vi "FUG_PowerSupply.ProcCases.vi"(0 "i ref in":refnum<vi>, 1 "selector":string, 2 "Data":T1, 3 "call cluster":T2={"Object"="", "Selector"="", "CallType"=enum."synchronous", "Async Object"="", "Async Selector"="", "Data Descriptor"="", "Data"=[], "Error #"=0, "Expire"=0}, 5 "error in (no error)":errorcluster) -> (14 "i ref out":refnum<vi>, 17 "answer cluster":T2={"Object"="", "Selector"="", "CallType"=enum."synchronous", "Async Object"="", "Async Selector"="", "Data Descriptor"="", "Data"=[], "Error #"=0, "Expire"=0}, 19 "error out":errorcluster)   [LabVIEW 2014, in "FUG_PowerSupply.lvlib"]
doc: "This method is called by a process from within the default case in the event loop. The methods of a class that are linked to events will be called from THIS method. Add your code here."
uses:
  FUG_PowerSupply.lvlib
  CS_Core/CSSystem/CoreDefs/CoreDefs.call_type.ctl
  CS_Core/BaseProcess/BaseProcess.descriptor string definition.ctl
  CS_Core/CSSystem/CoreDefs/CoreDefs.rawDataType.ctl
  CS_Core/CSSystem/CoreLib/CoreLib.byte array 2 short.vi
  CS_Core/CSSystem/CoreLib/CoreLib.byte array 2 int.vi
  CS_Core/CSSystem/CoreLib/CoreLib.string 2 byte array.vi
  CS_Core/CSSystem/CoreLib/CoreLib.byte array 2 double.vi
  CS_Core/CSSystem/CoreLib/CoreLib.lvlib
  CS_Core/BaseProcess/BaseProcess.lvlib
  CS_Core/CAEObj/CAEObj.lvlib
  CS_Core/CSApplicationBaseClasses/PSChannelBase/PSChannelBase.lvlib
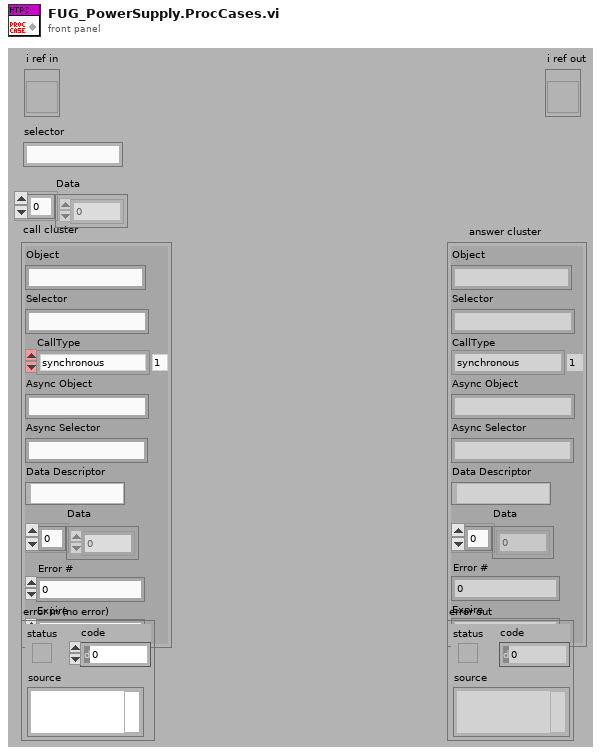
[diagram p1: front panel]
types:
  T1 = typedef "CoreDefs.rawDataType.ctl" = i8[]
  T2 = typedef "CoreDefs.call_type.ctl" = cluster{"Object":string, "Selector":string, "CallType":enum16{"simple", "synchronous", "asynchronous"}, "Async Object":string, "Async Selector":string, "Data Descriptor":T3, "Data":T1, "Error #":i32, "Expire":u32}
  T3 = typedef "BaseProcess.lvlib/BaseProcess.descriptor string definition.ctl" = string
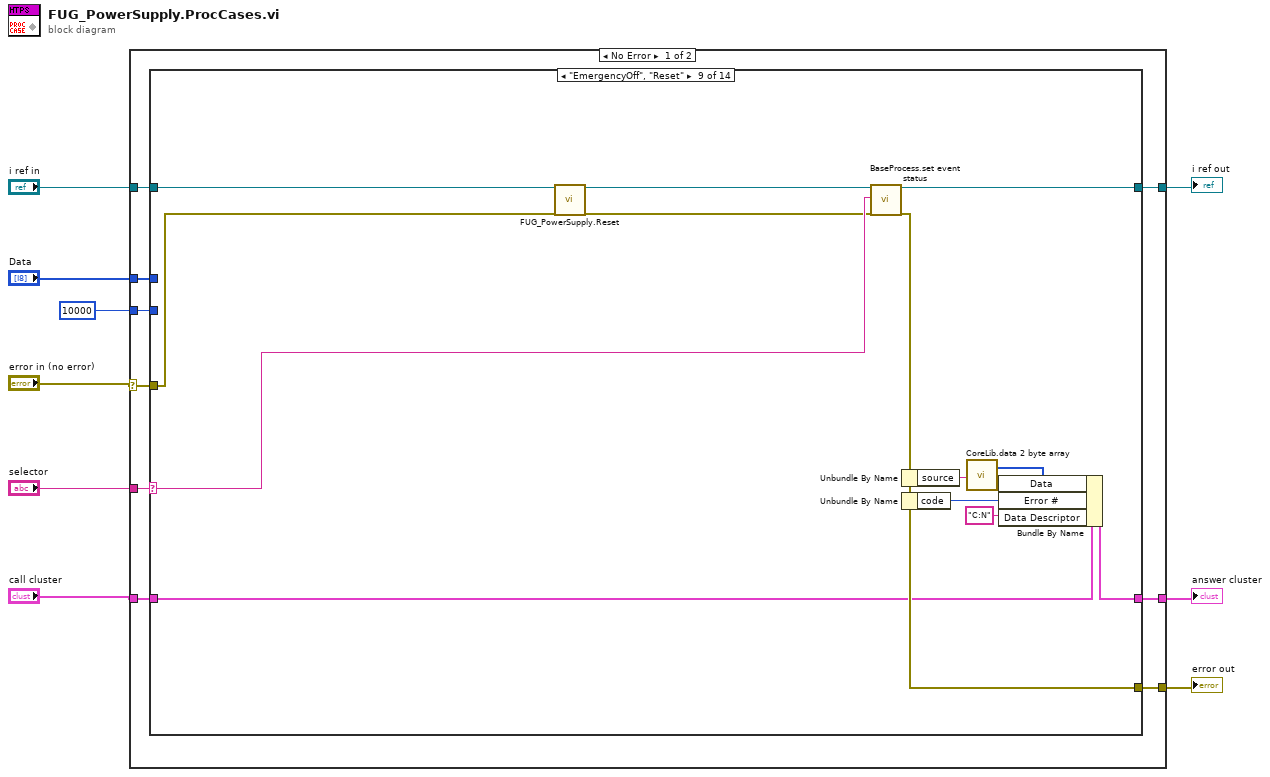
[diagram p0: block diagram]
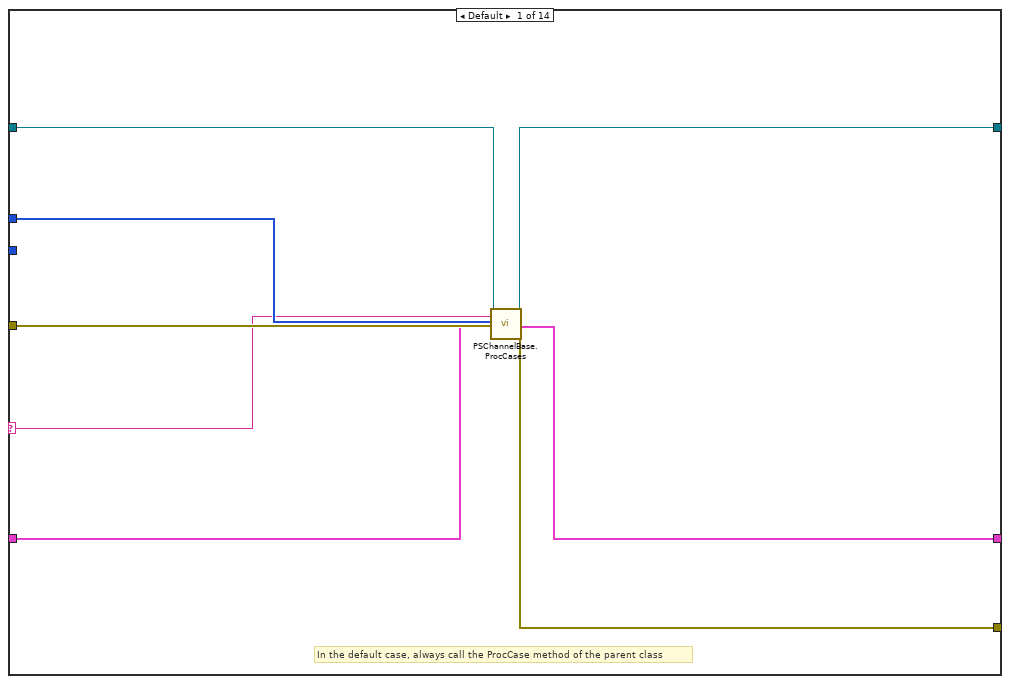
[diagram p2: hidden frame]
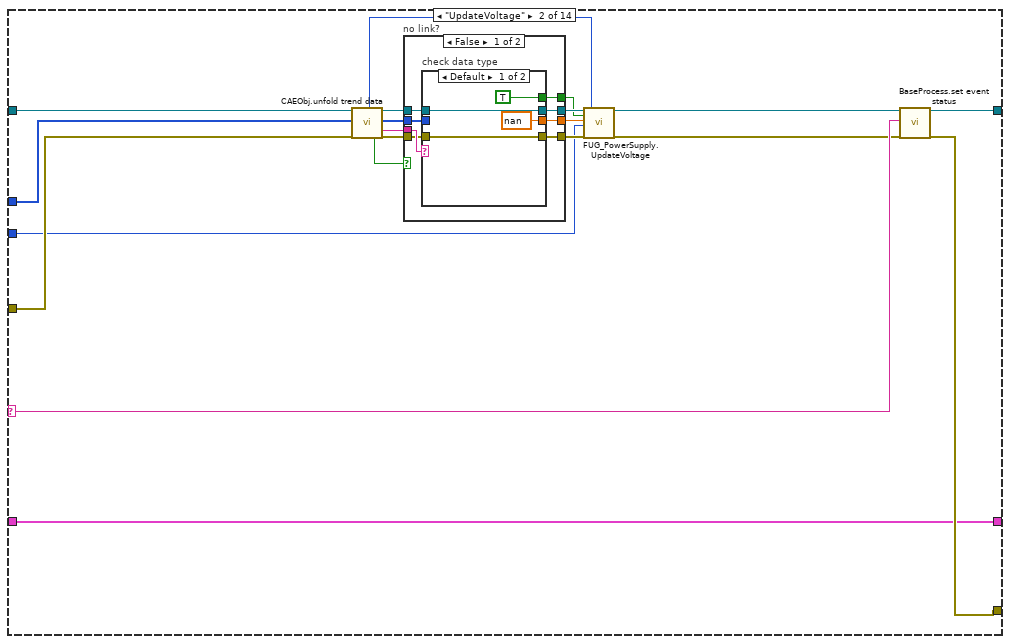
[diagram p3: hidden frame]
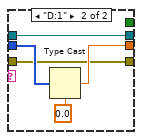
[diagram p4: hidden frame]
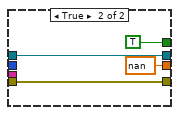
[diagram p5: hidden frame]
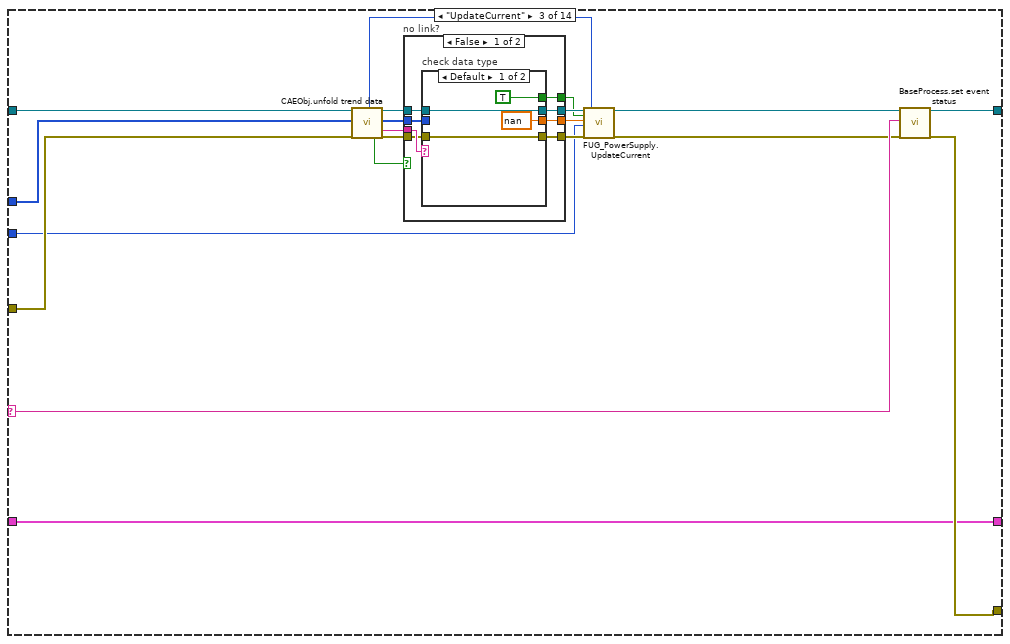
[diagram p6: hidden frame]
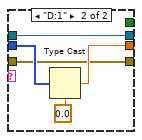
[diagram p7: hidden frame]
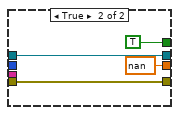
[diagram p8: hidden frame]
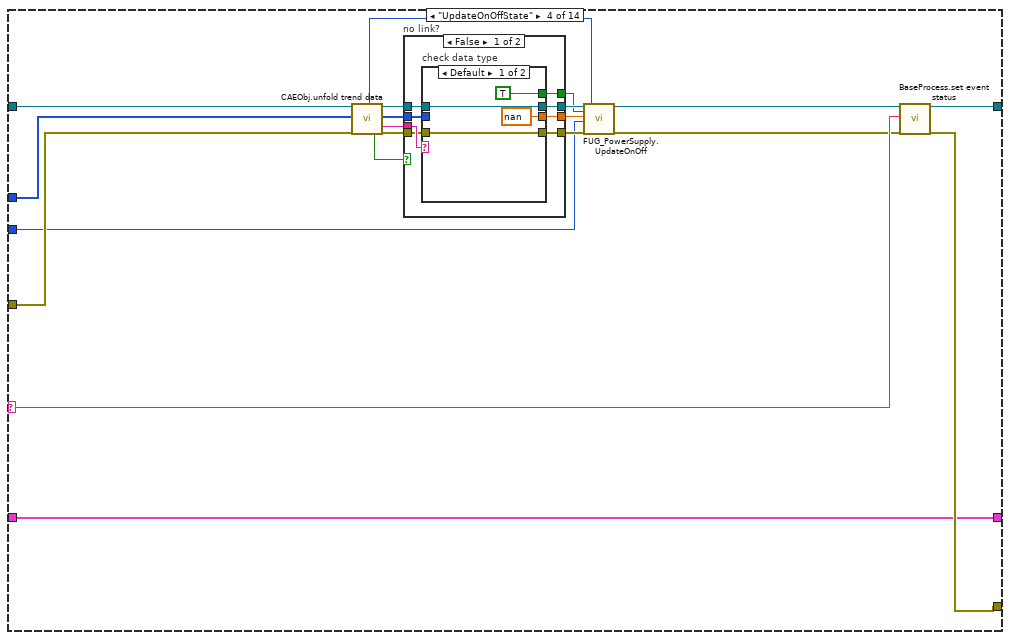
[diagram p9: hidden frame]
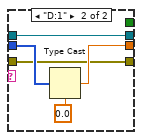
[diagram p10: hidden frame]
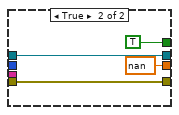
[diagram p11: hidden frame]
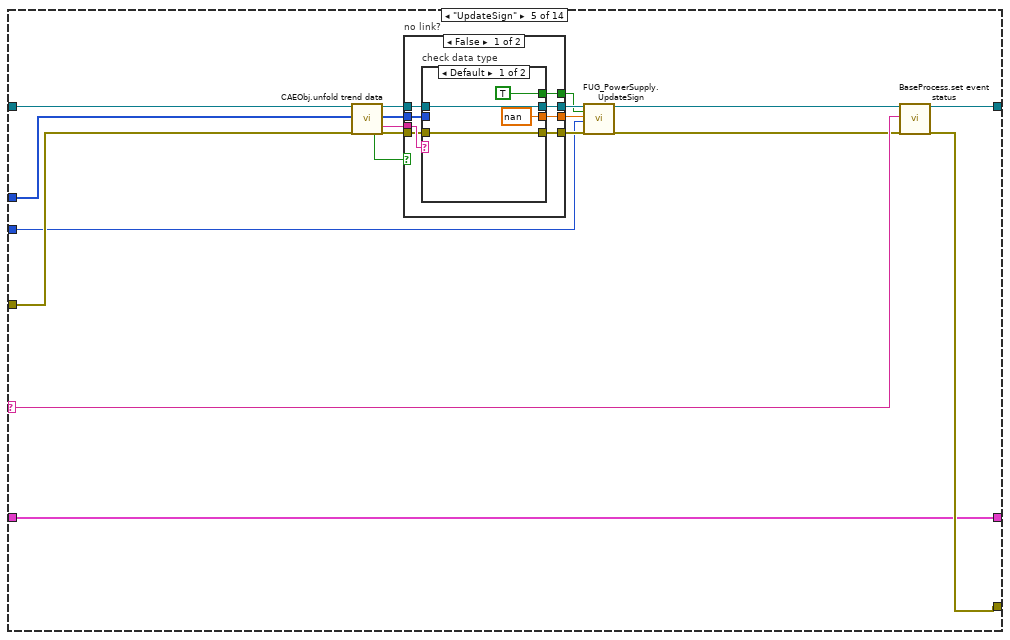
[diagram p12: hidden frame]
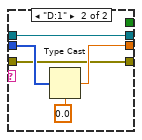
[diagram p13: hidden frame]
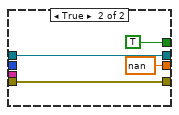
[diagram p14: hidden frame]
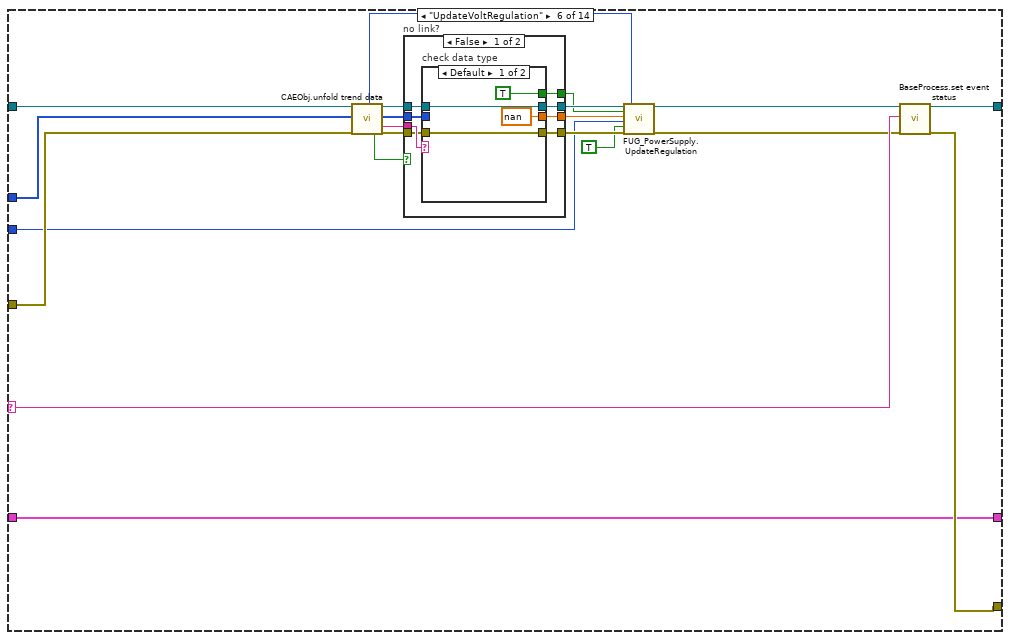
[diagram p15: hidden frame]
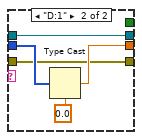
[diagram p16: hidden frame]
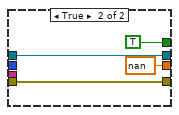
[diagram p17: hidden frame]
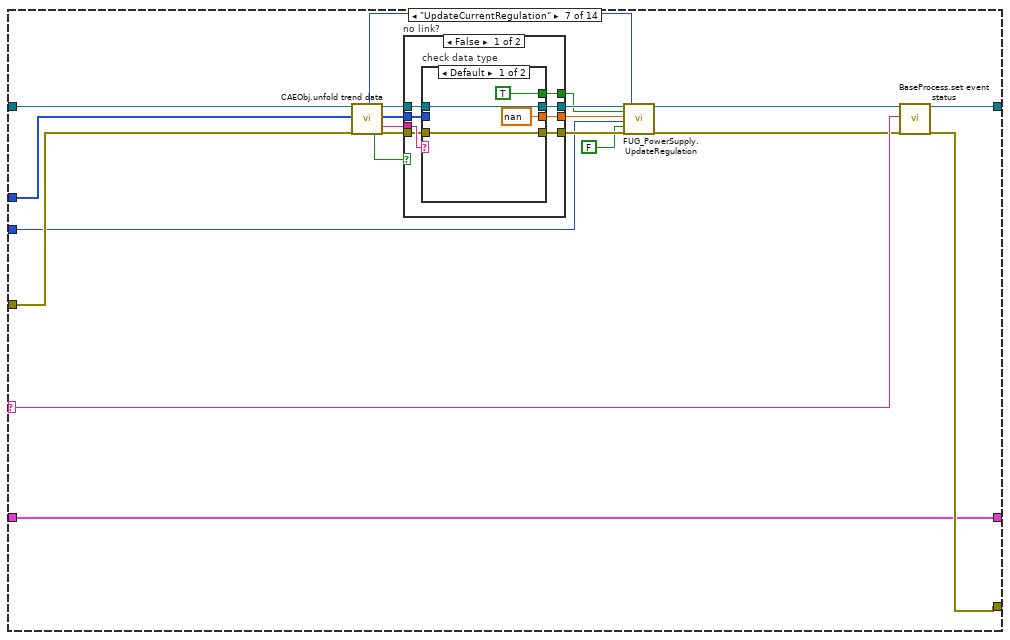
[diagram p18: hidden frame]
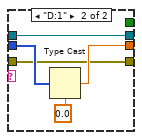
[diagram p19: hidden frame]
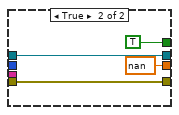
[diagram p20: hidden frame]
diagram:
  n1 = case shown="No Error" "error in (no error)" {
    selector: "error in (no error)" -> [w11 w453]
    tunnel: "selector" -> [w18 _]
    tunnel: [w17 w454] -> w3
    tunnel: "Data" -> [w16 _]
    tunnel: "call cluster" -> [w15 w454]
    tunnel: "i ref in" -> [w14 w455]
    tunnel: [w13 w455] -> w4
    tunnel: [w12 w453] -> w2
    tunnel: 10000 ("ms timeout (100)") -> [w10 _]
    frame No Error {
      n2 = case shown="\"EmergencyOff\", \"Reset\"" w18 {
        selector: w18 -> [w20 w40 w81 w122 w162 w204 w246 w285 w310 w328 w356 w386 w409 w435]
        tunnel: w16 -> [w21 w41 w82 w123 w163 w205 w247 _ _ _ _ _ _ _]
        tunnel: w14 -> [w19 w43 w84 w125 w165 w207 w249 w289 w312 w332 w360 w390 w411 w437]
        tunnel: [w26 w45 w86 w127 w167 w209 w251 w290 w313 w333 w361 w391 w414 w440] -> w13
        tunnel: w15 -> [w22 w44 w85 w126 w166 w208 w250 w277 w302 w321 w346 w377 w406 w433]
        tunnel: [w23 w44 w85 w126 w166 w208 w250 w280 w304 w323 w351 w381 w406 w433] -> w17
        tunnel: w11 -> [w25 w42 w83 w124 w164 w206 w248 w274 w301 w318 w345 w376 w403 w430]
        tunnel: [w24 w46 w87 w128 w168 w210 w252 w279 w303 w322 w350 w380 w413 w439] -> w12
        tunnel: w10 -> [_ w27 w68 w109 w150 w192 w234 _ _ _ _ _ _ _]
        frame Default {
          # "In the default case, always call the ProcCase method of the parent class"
          n3 = call "PSChannelBase.ProcCases.vi"("i ref in"=w19, "selector"=w20, "Data"=w21, "call cluster"=w22, "error in (no error)"=w25) -> ("i ref out"=w26:refnum<vi>, "answer cluster"=w23:T2, "error out"=w24:errorcluster)  [unwired: 12 in]
        }
        frame "UpdateVoltage" {
          n4 = call "CAEObj.unfold trend data.vi"("i ref in"=w43, "raw trend data"=w41, "error in (no error)"=w42) -> ("quality"=w28:i32, "no link"=w35:bool, "i ref out"=w39:refnum<vi>, "data"=w37:i8[], "typeDescriptor"=w36:string, "error out"=w38:errorcluster)  [unwired: 8 in, 3 out]
          n5 = case "no link?" shown="False" w35 {
            tunnel: [w54 w66] -> w34
            tunnel: [w53 w65] -> w33
            tunnel: w37 -> [w52 _]
            tunnel: w39 -> [w51 w66]
            tunnel: w36 -> [w50 _]
            tunnel: w38 -> [w49 w65]
            tunnel: [w48 TRUE ("badValue")] -> w30
            tunnel: [w47 nan] -> w29
            frame False {
              n6 = case "check data type" shown="Default" w50 {
                tunnel: [w56 w59] -> w54
                tunnel: [w57 w60] -> w53
                tunnel: w52 -> [_ w63]
                tunnel: w51 -> [w56 w59]
                tunnel: w49 -> [w57 w60]
                tunnel: [TRUE ("badValue") _] -> w48
                tunnel: [nan w61] -> w47
                frame Default {
                }
                frame "D:1" {
                  n7 = Type Cast(type=0.0, x=w63) -> (*(type *) &x=w61:dbl)
                }
              }
            }
            frame True {
            }
          }
          n8 = call "FUG_PowerSupply.UpdateVoltage.vi"("i ref in"=w34, "badValue"=w30, "moduleValue"=w29, "ms timeout (10000)"=w27, "error in (no error)"=w33, "voltageQuality"=w28) -> ("i ref out"=w32:refnum<vi>, "error out"=w31:errorcluster)  [unwired: 11 in, 1 out]
          n9 = call "BaseProcess.set event status.vi"("i ref in"=w32, "EventStatus"=w40, "error in (no error)"=w31) -> ("i ref out"=w45:refnum<vi>, "error out"=w46:errorcluster)  [unwired: 14 in, 1 out]
        }
        frame "UpdateCurrent" {
          n10 = call "CAEObj.unfold trend data.vi"("i ref in"=w84, "raw trend data"=w82, "error in (no error)"=w83) -> ("quality"=w69:i32, "no link"=w76:bool, "i ref out"=w80:refnum<vi>, "data"=w78:i8[], "typeDescriptor"=w77:string, "error out"=w79:errorcluster)  [unwired: 8 in, 3 out]
          n11 = case "no link?" shown="False" w76 {
            tunnel: [w95 w107] -> w75
            tunnel: [w94 w106] -> w74
            tunnel: w78 -> [w93 _]
            tunnel: w80 -> [w92 w107]
            tunnel: w77 -> [w91 _]
            tunnel: w79 -> [w90 w106]
            tunnel: [w89 TRUE ("badValue")] -> w71
            tunnel: [w88 nan] -> w70
            frame False {
              n12 = case "check data type" shown="Default" w91 {
                tunnel: [w97 w100] -> w95
                tunnel: [w98 w101] -> w94
                tunnel: w93 -> [_ w104]
                tunnel: w92 -> [w97 w100]
                tunnel: w90 -> [w98 w101]
                tunnel: [TRUE ("badValue") _] -> w89
                tunnel: [nan w102] -> w88
                frame Default {
                }
                frame "D:1" {
                  n13 = Type Cast(type=0.0, x=w104) -> (*(type *) &x=w102:dbl)
                }
              }
            }
            frame True {
            }
          }
          n14 = call "FUG_PowerSupply.UpdateCurrent.vi"("i ref in"=w75, "badValue"=w71, "moduleValue"=w70, "ms timeout (10000)"=w68, "error in (no error)"=w74, "quality"=w69) -> ("i ref out"=w73:refnum<vi>, "error out"=w72:errorcluster)  [unwired: 11 in, 1 out]
          n15 = call "BaseProcess.set event status.vi"("i ref in"=w73, "EventStatus"=w81, "error in (no error)"=w72) -> ("i ref out"=w86:refnum<vi>, "error out"=w87:errorcluster)  [unwired: 14 in, 1 out]
        }
        frame "UpdateOnOffState" {
          n16 = call "CAEObj.unfold trend data.vi"("i ref in"=w125, "raw trend data"=w123, "error in (no error)"=w124) -> ("quality"=w110:i32, "no link"=w117:bool, "i ref out"=w121:refnum<vi>, "data"=w119:i8[], "typeDescriptor"=w118:string, "error out"=w120:errorcluster)  [unwired: 8 in, 3 out]
          n17 = case "no link?" shown="False" w117 {
            tunnel: [w136 w148] -> w116
            tunnel: [w135 w147] -> w115
            tunnel: w119 -> [w134 _]
            tunnel: w121 -> [w133 w148]
            tunnel: w118 -> [w132 _]
            tunnel: w120 -> [w131 w147]
            tunnel: [w130 TRUE ("badValue")] -> w112
            tunnel: [w129 nan] -> w111
            frame False {
              n18 = case "check data type" shown="Default" w132 {
                tunnel: [w138 w141] -> w136
                tunnel: [w139 w142] -> w135
                tunnel: w134 -> [_ w145]
                tunnel: w133 -> [w138 w141]
                tunnel: w131 -> [w139 w142]
                tunnel: [TRUE ("badValue") _] -> w130
                tunnel: [nan w143] -> w129
                frame Default {
                }
                frame "D:1" {
                  n19 = Type Cast(type=0.0, x=w145) -> (*(type *) &x=w143:dbl)
                }
              }
            }
            frame True {
            }
          }
          n20 = call "FUG_PowerSupply.UpdateOnOff.vi"("i ref in"=w116, "badValue"=w112, "moduleValue"=w111, "ms timeout (10000)"=w109, "error in (no error)"=w115, "onOffQuality"=w110) -> ("i ref out"=w114:refnum<vi>, "error out"=w113:errorcluster)  [unwired: 11 in, 1 out]
          n21 = call "BaseProcess.set event status.vi"("i ref in"=w114, "EventStatus"=w122, "error in (no error)"=w113) -> ("i ref out"=w127:refnum<vi>, "error out"=w128:errorcluster)  [unwired: 14 in, 1 out]
        }
        frame "UpdateSign" {
          n22 = call "CAEObj.unfold trend data.vi"("i ref in"=w165, "raw trend data"=w163, "error in (no error)"=w164) -> ("no link"=w157:bool, "i ref out"=w161:refnum<vi>, "data"=w159:i8[], "typeDescriptor"=w158:string, "error out"=w160:errorcluster)  [unwired: 8 in, 4 out]
          n23 = case "no link?" shown="False" w157 {
            tunnel: [w176 w188] -> w156
            tunnel: [w175 w187] -> w155
            tunnel: w159 -> [w174 _]
            tunnel: w161 -> [w173 w188]
            tunnel: w158 -> [w172 _]
            tunnel: w160 -> [w171 w187]
            tunnel: [w170 TRUE ("badValue")] -> w152
            tunnel: [w169 nan] -> w151
            frame False {
              n24 = case "check data type" shown="Default" w172 {
                tunnel: [w178 w181] -> w176
                tunnel: [w179 w182] -> w175
                tunnel: w174 -> [_ w185]
                tunnel: w173 -> [w178 w181]
                tunnel: w171 -> [w179 w182]
                tunnel: [TRUE ("badValue") _] -> w170
                tunnel: [nan w183] -> w169
                frame Default {
                }
                frame "D:1" {
                  n25 = Type Cast(type=0.0, x=w185) -> (*(type *) &x=w183:dbl)
                }
              }
            }
            frame True {
            }
          }
          n26 = call "FUG_PowerSupply.UpdateSign.vi"("i ref in"=w156, "badValue"=w152, "moduleValue"=w151, "ms timeout (10000)"=w150, "error in (no error)"=w155) -> ("i ref out"=w154:refnum<vi>, "error out"=w153:errorcluster)  [unwired: 12 in, 1 out]
          n27 = call "BaseProcess.set event status.vi"("i ref in"=w154, "EventStatus"=w162, "error in (no error)"=w153) -> ("i ref out"=w167:refnum<vi>, "error out"=w168:errorcluster)  [unwired: 14 in, 1 out]
        }
        frame "UpdateVoltRegulation" {
          n28 = call "CAEObj.unfold trend data.vi"("i ref in"=w207, "raw trend data"=w205, "error in (no error)"=w206) -> ("quality"=w191:i32, "no link"=w199:bool, "i ref out"=w203:refnum<vi>, "data"=w201:i8[], "typeDescriptor"=w200:string, "error out"=w202:errorcluster)  [unwired: 8 in, 3 out]
          n29 = case "no link?" shown="False" w199 {
            tunnel: [w218 w230] -> w198
            tunnel: [w217 w229] -> w197
            tunnel: w201 -> [w216 _]
            tunnel: w203 -> [w215 w230]
            tunnel: w200 -> [w214 _]
            tunnel: w202 -> [w213 w229]
            tunnel: [w212 TRUE ("badValue")] -> w194
            tunnel: [w211 nan] -> w193
            frame False {
              n30 = case "check data type" shown="Default" w214 {
                tunnel: [w220 w223] -> w218
                tunnel: [w221 w224] -> w217
                tunnel: w216 -> [_ w227]
                tunnel: w215 -> [w220 w223]
                tunnel: w213 -> [w221 w224]
                tunnel: [TRUE ("badValue") _] -> w212
                tunnel: [nan w225] -> w211
                frame Default {
                }
                frame "D:1" {
                  n31 = Type Cast(type=0.0, x=w227) -> (*(type *) &x=w225:dbl)
                }
              }
            }
            frame True {
            }
          }
          n32 = call "FUG_PowerSupply.UpdateRegulation.vi"("i ref in"=w198, "badValue"=w194, "moduleValue"=w193, "ms timeout (10000)"=w192, "voltageRegulation"=TRUE, "error in (no error)"=w197, "valueQuality"=w191) -> ("i ref out"=w196:refnum<vi>, "error out"=w195:errorcluster)  [unwired: 10 in, 1 out]
          n33 = call "BaseProcess.set event status.vi"("i ref in"=w196, "EventStatus"=w204, "error in (no error)"=w195) -> ("i ref out"=w209:refnum<vi>, "error out"=w210:errorcluster)  [unwired: 14 in, 1 out]
        }
        frame "UpdateCurrentRegulation" {
          n34 = call "CAEObj.unfold trend data.vi"("i ref in"=w249, "raw trend data"=w247, "error in (no error)"=w248) -> ("quality"=w233:i32, "no link"=w241:bool, "i ref out"=w245:refnum<vi>, "data"=w243:i8[], "typeDescriptor"=w242:string, "error out"=w244:errorcluster)  [unwired: 8 in, 3 out]
          n35 = case "no link?" shown="False" w241 {
            tunnel: [w260 w272] -> w240
            tunnel: [w259 w271] -> w239
            tunnel: w243 -> [w258 _]
            tunnel: w245 -> [w257 w272]
            tunnel: w242 -> [w256 _]
            tunnel: w244 -> [w255 w271]
            tunnel: [w254 TRUE ("badValue")] -> w236
            tunnel: [w253 nan] -> w235
            frame False {
              n36 = case "check data type" shown="Default" w256 {
                tunnel: [w262 w265] -> w260
                tunnel: [w263 w266] -> w259
                tunnel: w258 -> [_ w269]
                tunnel: w257 -> [w262 w265]
                tunnel: w255 -> [w263 w266]
                tunnel: [TRUE ("badValue") _] -> w254
                tunnel: [nan w267] -> w253
                frame Default {
                }
                frame "D:1" {
                  n37 = Type Cast(type=0.0, x=w269) -> (*(type *) &x=w267:dbl)
                }
              }
            }
            frame True {
            }
          }
          n38 = call "FUG_PowerSupply.UpdateRegulation.vi"("i ref in"=w240, "badValue"=w236, "moduleValue"=w235, "ms timeout (10000)"=w234, "voltageRegulation"=FALSE, "error in (no error)"=w239, "valueQuality"=w233) -> ("i ref out"=w238:refnum<vi>, "error out"=w237:errorcluster)  [unwired: 10 in, 1 out]
          n39 = call "BaseProcess.set event status.vi"("i ref in"=w238, "EventStatus"=w246, "error in (no error)"=w237) -> ("i ref out"=w251:refnum<vi>, "error out"=w252:errorcluster)  [unwired: 14 in, 1 out]
        }
        frame "SetCurrent" {
          n40 = Unbundle By Name(w277) -> ("Data"=w278:T1)
          n41 = call-poly "CoreLib.byte array 2 data.vi"("byteArray"=w278) -> ("d64"=w275:dbl, "error out"=w276:errorcluster)  [unwired: 16 in, 1 out]
          n42 = case shown="No Error" w276 {
            selector: w276 -> [_ w300]
            tunnel: w285 -> [w292 w299]
            tunnel: [w292 w299] -> w287
            tunnel: [w294 w298] -> w286
            tunnel: w289 -> [w296 w297]
            tunnel: [w295 w297] -> w288
            tunnel: w275 -> [w291 _]
            tunnel: w274 -> [w293 _]
            frame No Error {
              n43 = call "FUG_PowerSupply.SetCurrent.vi"("i ref in"=w296, "value"=w291, "error in (no error)"=w293) -> ("i ref out"=w295:refnum<vi>, "error out (no error)"=w294:errorcluster)  [unwired: 15 in]
            }
            frame Error {
              n44 = call "CoreLib.set data type mismatch.vi"("error in (no error)"=w300, "error source"=w299) -> ("error out"=w298:errorcluster)  [unwired: 17 in]
            }
          }
          n45 = call "BaseProcess.set event status.vi"("i ref in"=w288, "EventStatus"=w287, "error in (no error)"=w286) -> ("i ref out"=w290:refnum<vi>, "error out"=w279:errorcluster)  [unwired: 14 in, 1 out]
          n46 = Unbundle By Name(w279) -> ("source"=w281:string)
          n47 = Unbundle By Name(w279) -> ("code"=w284:i32)
          n48 = call-poly "CoreLib.data 2 byte array.vi"("string"=w281) -> ("byteArray out"=w283:T1)  [unwired: 18 in]
          n49 = Bundle By Name(cluster=w277, "Data"=w283, "Error #"=w284, "Data Descriptor"="C:N") -> (w280:T2)
        }
        frame "EmergencyOff", "Reset" {
          n50 = call "FUG_PowerSupply.Reset.vi"("i ref in"=w312, "error in (no error)"=w301) -> ("i ref out"=w311:refnum<vi>, "error out (no error)"=w309:errorcluster)  [unwired: 16 in]
          n51 = call "BaseProcess.set event status.vi"("i ref in"=w311, "EventStatus"=w310, "error in (no error)"=w309) -> ("i ref out"=w313:refnum<vi>, "error out"=w303:errorcluster)  [unwired: 14 in, 1 out]
          n52 = Unbundle By Name(w303) -> ("source"=w305:string)
          n53 = Unbundle By Name(w303) -> ("code"=w308:i32)
          n54 = call-poly "CoreLib.data 2 byte array.vi"("string"=w305) -> ("byteArray out"=w307:T1)  [unwired: 18 in]
          n55 = Bundle By Name(cluster=w302, "Data"=w307, "Error #"=w308, "Data Descriptor"="C:N") -> (w304:T2)
        }
        frame "SetChannelCurrent" {
          n56 = Unbundle By Name(w321) -> ("Data"=w317:T1)
          n57 = call-poly "CoreLib.byte array 2 data.vi"("byteArray"=w317) -> ("byteArray out"=w316:T1, "i32"=w314:i32, "error out"=w315:errorcluster)  [unwired: 16 in]
          n58 = call-poly "CoreLib.byte array 2 data.vi"("byteArray"=w316, "error in (no error)"=w315) -> ("d64"=w319:dbl, "error out"=w320:errorcluster)  [unwired: 15 in, 1 out]
          n59 = case shown="No Error" w320 {
            selector: w320 -> [_ w344]
            tunnel: w328 -> [w336 w343]
            tunnel: [w336 w343] -> w330
            tunnel: [w338 w342] -> w329
            tunnel: w332 -> [w340 w341]
            tunnel: [w339 w341] -> w331
            tunnel: w319 -> [w335 _]
            tunnel: w318 -> [w337 _]
            tunnel: w314 -> [w334 _]
            frame No Error {
              n60 = call "FUG_PowerSupply.SetCurrent.vi"("i ref in"=w340, "value"=w335, "error in (no error)"=w337, "channel"=w334) -> ("i ref out"=w339:refnum<vi>, "error out (no error)"=w338:errorcluster)  [unwired: 14 in]
            }
            frame Error {
              n61 = call "CoreLib.set data type mismatch.vi"("error in (no error)"=w344, "error source"=w343) -> ("error out"=w342:errorcluster)  [unwired: 17 in]
            }
          }
          n62 = call "BaseProcess.set event status.vi"("i ref in"=w331, "EventStatus"=w330, "error in (no error)"=w329) -> ("i ref out"=w333:refnum<vi>, "error out"=w322:errorcluster)  [unwired: 14 in, 1 out]
          n63 = Unbundle By Name(w322) -> ("source"=w324:string)
          n64 = Unbundle By Name(w322) -> ("code"=w327:i32)
          n65 = call-poly "CoreLib.data 2 byte array.vi"("string"=w324) -> ("byteArray out"=w326:T1)  [unwired: 18 in]
          n66 = Bundle By Name(cluster=w321, "Data"=w326, "Error #"=w327, "Data Descriptor"="C:N") -> (w323:T2)
        }
        frame "SetVoltage" {
          n67 = Unbundle By Name(w346) -> ("Data"=w349:T1)
          n68 = call-poly "CoreLib.byte array 2 data.vi"("byteArray"=w349) -> ("d64"=w347:dbl, "error out"=w348:errorcluster)  [unwired: 16 in, 1 out]
          n69 = case shown="No Error" w348 {
            selector: w348 -> [_ w371]
            tunnel: w356 -> [w364 w370]
            tunnel: [w364 w370] -> w358
            tunnel: [w365 w369] -> w357
            tunnel: w360 -> [w367 w368]
            tunnel: [w366 w368] -> w359
            tunnel: w347 -> [w363 _]
            tunnel: w345 -> [w362 _]
            frame No Error {
              n70 = call "FUG_PowerSupply.SetVoltage.vi"("i ref in"=w367, "value"=w363, "error in (no error)"=w362) -> ("i ref out"=w366:refnum<vi>, "error out (no error)"=w365:errorcluster)  [unwired: 15 in]
            }
            frame Error {
              n71 = call "CoreLib.set data type mismatch.vi"("error in (no error)"=w371, "error source"=w370) -> ("error out"=w369:errorcluster)  [unwired: 17 in]
            }
          }
          n72 = call "BaseProcess.set event status.vi"("i ref in"=w359, "EventStatus"=w358, "error in (no error)"=w357) -> ("i ref out"=w361:refnum<vi>, "error out"=w350:errorcluster)  [unwired: 14 in, 1 out]
          n73 = Unbundle By Name(w350) -> ("source"=w352:string)
          n74 = Unbundle By Name(w350) -> ("code"=w355:i32)
          n75 = call-poly "CoreLib.data 2 byte array.vi"("string"=w352) -> ("byteArray out"=w354:T1)  [unwired: 18 in]
          n76 = Bundle By Name(cluster=w346, "Data"=w354, "Error #"=w355, "Data Descriptor"="C:N") -> (w351:T2)
        }
        frame "SetChannelVoltage" {
          n77 = Unbundle By Name(w377) -> ("Data"=w375:T1)
          n78 = call-poly "CoreLib.byte array 2 data.vi"("byteArray"=w375) -> ("byteArray out"=w373:T1, "i32"=w372:i32, "error out"=w374:errorcluster)  [unwired: 16 in]
          n79 = call-poly "CoreLib.byte array 2 data.vi"("byteArray"=w373, "error in (no error)"=w374) -> ("d64"=w378:dbl, "error out"=w379:errorcluster)  [unwired: 15 in, 1 out]
          n80 = case shown="No Error" w379 {
            selector: w379 -> [_ w402]
            tunnel: w386 -> [w395 w401]
            tunnel: [w395 w401] -> w388
            tunnel: [w396 w400] -> w387
            tunnel: w390 -> [w398 w399]
            tunnel: [w397 w399] -> w389
            tunnel: w378 -> [w394 _]
            tunnel: w376 -> [w393 _]
            tunnel: w372 -> [w392 _]
            frame No Error {
              n81 = call "FUG_PowerSupply.SetVoltage.vi"("i ref in"=w398, "value"=w394, "error in (no error)"=w393, "channelIndex"=w392) -> ("i ref out"=w397:refnum<vi>, "error out (no error)"=w396:errorcluster)  [unwired: 14 in]
            }
            frame Error {
              n82 = call "CoreLib.set data type mismatch.vi"("error in (no error)"=w402, "error source"=w401) -> ("error out"=w400:errorcluster)  [unwired: 17 in]
            }
          }
          n83 = call "BaseProcess.set event status.vi"("i ref in"=w389, "EventStatus"=w388, "error in (no error)"=w387) -> ("i ref out"=w391:refnum<vi>, "error out"=w380:errorcluster)  [unwired: 14 in, 1 out]
          n84 = Unbundle By Name(w380) -> ("source"=w382:string)
          n85 = Unbundle By Name(w380) -> ("code"=w385:i32)
          n86 = call-poly "CoreLib.data 2 byte array.vi"("string"=w382) -> ("byteArray out"=w384:T1)  [unwired: 18 in]
          n87 = Bundle By Name(cluster=w377, "Data"=w384, "Error #"=w385, "Data Descriptor"="C:N") -> (w381:T2)
        }
        frame "SetOnOff" {
          n88 = Unbundle By Name(w406) -> ("Data"=w407:T1)
          n89 = call-poly "CoreLib.byte array 2 data.vi"("byteArray"=w407) -> ("i16"=w405:i16, "error out"=w404:errorcluster)  [unwired: 16 in, 1 out]
          n90 = case shown="No Error" w404 {
            selector: w404 -> [_ w425]
            tunnel: w409 -> [w421 w424]
            tunnel: [w421 w424] -> w410
            tunnel: [w416 w423] -> w408
            tunnel: w411 -> [w420 w422]
            tunnel: [w419 w422] -> w412
            tunnel: w405 -> [w418 _]
            tunnel: w403 -> [w415 _]
            frame No Error {
              n91 = Greater Than 0?(x=w418) -> (x > 0?=w417:bool)
              n92 = call "FUG_PowerSupply.SetOnOff.vi"("i ref in"=w420, "value"=w417, "error in (no error)"=w415) -> ("i ref out"=w419:refnum<vi>, "error out (no error)"=w416:errorcluster)  [unwired: 15 in]
            }
            frame Error {
              n93 = call "CoreLib.set data type mismatch.vi"("error in (no error)"=w425, "error source"=w424) -> ("error out"=w423:errorcluster)  [unwired: 17 in]
            }
          }
          n94 = call "BaseProcess.set event status.vi"("i ref in"=w412, "EventStatus"=w410, "error in (no error)"=w408) -> ("i ref out"=w414:refnum<vi>, "error out"=w413:errorcluster)  [unwired: 14 in, 1 out]
        }
        frame "SetChannelOnOff" {
          n95 = Unbundle By Name(w433) -> ("Data"=w429:T1)
          n96 = call-poly "CoreLib.byte array 2 data.vi"("byteArray"=w429) -> ("byteArray out"=w428:T1, "i32"=w426:i32, "error out"=w427:errorcluster)  [unwired: 16 in]
          n97 = call-poly "CoreLib.byte array 2 data.vi"("byteArray"=w428, "error in (no error)"=w427) -> ("i16"=w432:i16, "error out"=w431:errorcluster)  [unwired: 15 in, 1 out]
          n98 = case shown="No Error" w431 {
            selector: w431 -> [_ w452]
            tunnel: w435 -> [w448 w451]
            tunnel: [w448 w451] -> w436
            tunnel: [w443 w450] -> w434
            tunnel: w437 -> [w447 w449]
            tunnel: [w446 w449] -> w438
            tunnel: w432 -> [w445 _]
            tunnel: w430 -> [w442 _]
            tunnel: w426 -> [w441 _]
            frame No Error {
              n99 = Greater Than 0?(x=w445) -> (x > 0?=w444:bool)
              n100 = call "FUG_PowerSupply.SetOnOff.vi"("i ref in"=w447, "value"=w444, "error in (no error)"=w442, "channelIndex"=w441) -> ("i ref out"=w446:refnum<vi>, "error out (no error)"=w443:errorcluster)  [unwired: 14 in]
            }
            frame Error {
              n101 = call "CoreLib.set data type mismatch.vi"("error in (no error)"=w452, "error source"=w451) -> ("error out"=w450:errorcluster)  [unwired: 17 in]
            }
          }
          n102 = call "BaseProcess.set event status.vi"("i ref in"=w438, "EventStatus"=w436, "error in (no error)"=w434) -> ("i ref out"=w440:refnum<vi>, "error out"=w439:errorcluster)  [unwired: 14 in, 1 out]
        }
      }
    }
    frame Error {
    }
  }
  "answer cluster" <- w3
  "i ref out" <- w4
  "error out" <- w2
